vi "VSSDecodeFIRASimRobots.vi"(6 "FIRASim?":bool, 8 "error in":errorcluster, 9 "Time Stamp":timestamp, 10 "Robots":u8[](array[numeric]), 11 "Key":i32=5) -> (0 "error out":errorcluster, 2 "array w/ subset deleted out":u8[](array[numeric]), 3 "Robots":T1[](array[typedef]) {"height" format="%+4.3f"; "pixel_y" format="%+4.3f"; "pixel_x" format="%+4.3f"; "orientation" format="%+4.3f"; "y" format="%+4.3f"; "confidence" format="%4.3f"; "x" format="%+4.3f"})   [LabVIEW 2023]
uses:
  Controls/SSL Detection Robot.ctl
  <vilib>/Analysis/Matrix/Datatypes/RealMatrix.ctl
  <vilib>/Analysis/Matrix/NI_Matrix.lvlib
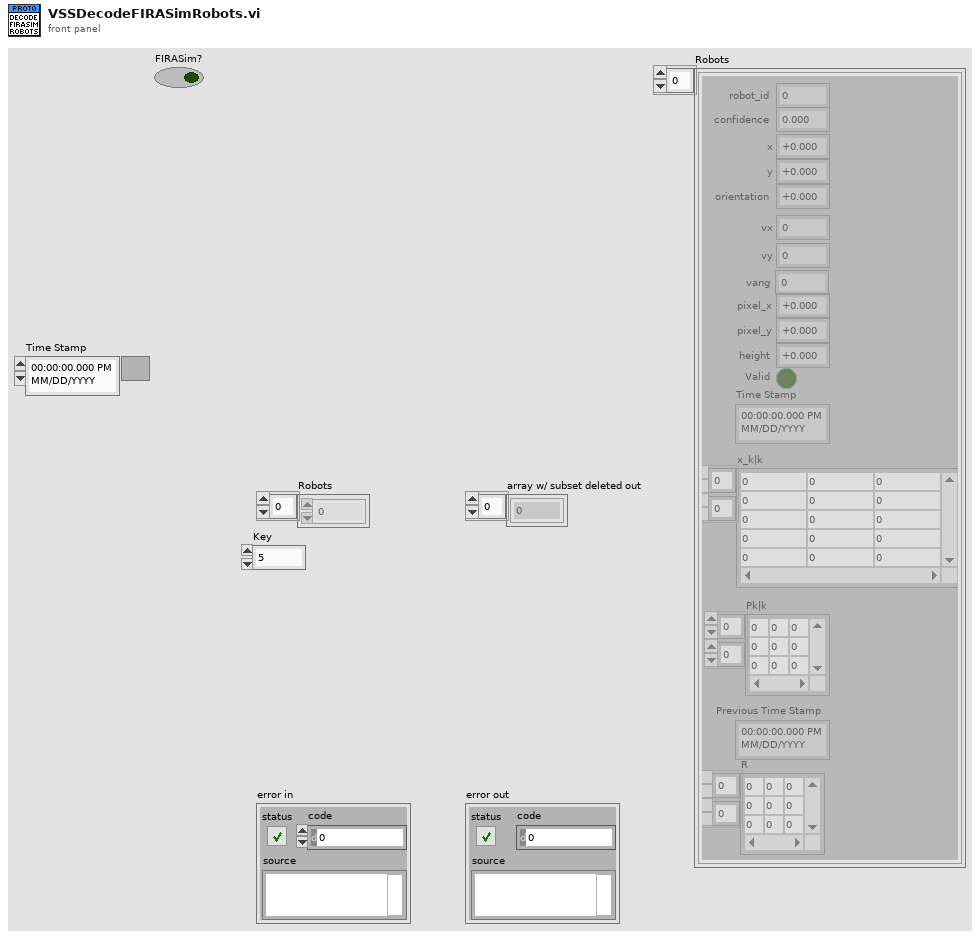
[diagram p1: front panel]
types:
  T1 = typedef "SSL Detection Robot.ctl" = cluster{"x":sgl, "robot_id":u32, "confidence":sgl, "y":sgl, "orientation":sgl, "pixel_x":sgl, "pixel_y":sgl, "height":sgl, "Valid":bool, "Time Stamp":timestamp, "x_k|k":T2, "Pk|k":T2, "Previous Time Stamp":timestamp, "R":T2, "vx":dbl, "vy":dbl, "vang":dbl}
  T2 = typedef "NI_Matrix.lvlib/RealMatrix.ctl" = dbl[][]
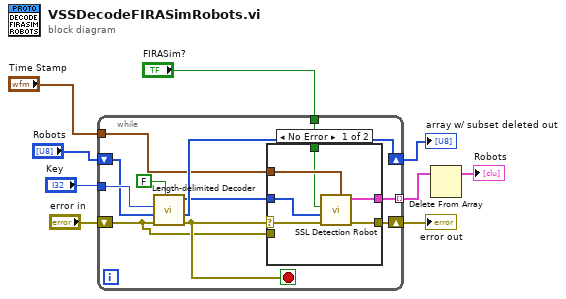
[diagram p0: block diagram]
diagram:
  n1 = while {
    shift-right: [w18] -> w7
    shift-left: "Robots" -> [w16]
    tunnel: [w20] -> w6 mode=indexing
    shift-right: [w19] -> w9
    shift-left: "error in" -> [w10]
    tunnel: "Key" -> [w17]
    tunnel: "Time Stamp" -> [w15]
    tunnel: "FIRASim?" -> [w14]
    stop <- w12 stop-if-true
    n2 = call "Length-delimited Decoder.vi"("Optional"=FALSE, "error in (no error)"=w10, "Array"=w16, "Key"=w17) -> ("error out"=w12:errorcluster, "array w/ subset deleted"=w18:u8[], "Length-delimited"=w13:u8[])  [unwired: 4 in, 1 out]
    n3 = case shown="No Error" w12 {
      selector: w12 -> [w21 _]
      tunnel: [w26 _] -> w20
      tunnel: [w25 w27] -> w19
      tunnel: w13 -> [w24 _]
      tunnel: w15 -> [w23 _]
      tunnel: w14 -> [w22 _]
      tunnel: w10 -> [_ w27]
      frame No Error {
        n4 = call "SSL Detection Robot.vi"("Time Stamp"=w23, "error in"=w21, "Robots"=w24, "FIRASim?"=w22) -> ("error out"=w25:errorcluster, "Detection Robot"=w26:T1)  [unwired: 5 in, 1 out]
      }
      frame Error {
      }
    }
  }
  "error out" <- w9
  "array w/ subset deleted out" <- w7
  n5 = Delete From Array(array=w6) -> (array with subset deleted=→"Robots":T1[])  [unwired: 2 in, 1 out]
